vi "Get Transparent buttons.vi"(8 "error in":errorcluster, 11 "Plain Parent in":refnum<class "Plain Parent.lvclass">) -> (0 "error out":errorcluster, 2 "Transparent buttons?":bool, 3 "Plain Parent out":refnum<class "Plain Parent.lvclass">)   [LabVIEW 2021, in "Pop-Up.lvlib" / "Plain Parent.lvclass"]
doc: "DATA MEMBER ACCESS:\n\nGet the transparent button Boolean info"
uses:
  Plain Parent.lvclass
  Plain Parent.lvclass/Plain Parent.ctl
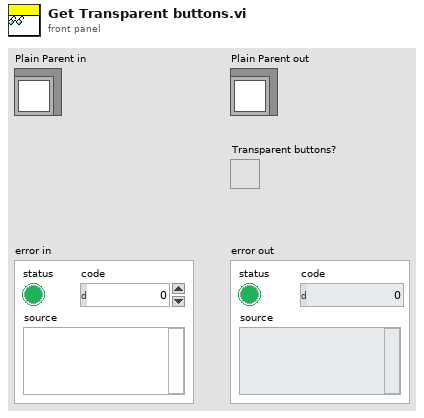
[diagram p1: front panel]
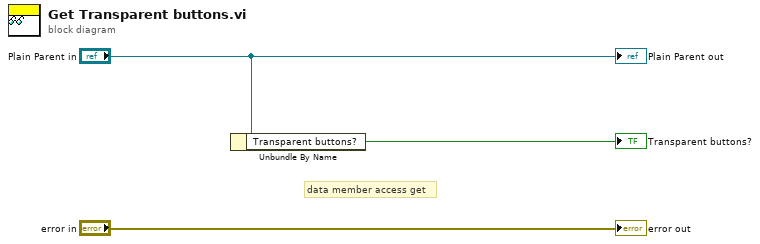
[diagram p0: block diagram]
diagram:
  # "data member access get"
  n1 = Unbundle By Name("Plain Parent in") -> ("Transparent buttons?"=→"Transparent buttons?":bool)
  "error out" <- "error in"
  "Plain Parent out" <- "Plain Parent in"
